vi "Magnet next action.vi"(4 "Overall status in":T2) -> (0 "Overall status Out":T2, 1 "Command out":T1=enum."Set field")   [LabVIEW 2024, in "Magnet module.lvlib"]
doc: "Evaluates next state machine action at the end of regular check.\nIf field is not at desired value, but reached the closest target it sets new target with new ramp."
uses:
  Magnet module.lvlib
  ctl/Overall status.ctl
  ctl/SetField data.ctl
  ctl/Magnet mode public.ctl
  ctl/Actual magnet state.ctl
  ctl/Magnet mode.ctl
  ctl/RampingOutput.ctl
  ctl/Magnet Orders.ctl
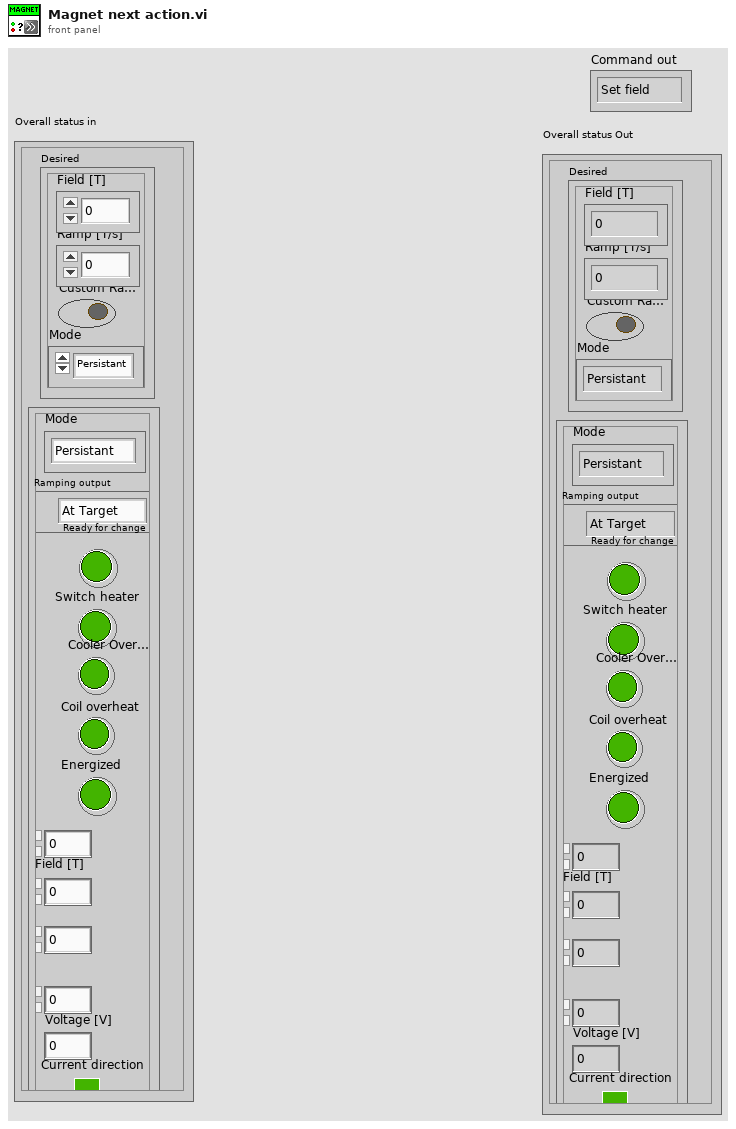
[diagram p1: front panel]
types:
  T1 = typedef "Magnet module.lvlib/Magnet Orders.ctl" = enum16{"Ignore", "Connect", "Update", "Switch mode", "Set field", "Stop ramping", "Equalize output", "Zero output", "Flip polarity", "Blackout", "Set timer", "Eval temperatures", "Disconnect"}
  T2 = typedef "Magnet module.lvlib/Overall status.ctl" = cluster{"Desired":T3, "Actual":T5}
  T3 = typedef "Magnet module.lvlib/SetField data.ctl" = cluster{"Field [T]":dbl, "Ramp [T/s]":dbl, "Custom Ramp?":bool, "Mode":T4}
  T4 = typedef "Magnet module.lvlib/Magnet mode public.ctl" = enum16{"Persistant", "Ramping"}
  T5 = typedef "Magnet module.lvlib/Actual magnet state.ctl" = cluster{"Mode":T6, "Ramping output":T7, "Ready for change":bool, "Switch heater":bool, "Cooler Overheat":bool, "Coil overheat":bool, "Energized":bool, "Output [T]":dbl, "Field [T]":dbl, "Ramp[T/s]":dbl, "Switch\ntemperature [K]":dbl, "Voltage [V]":dbl, "Current direction":bool}
  T6 = typedef "Magnet module.lvlib/Magnet mode.ctl" = enum16{"Persistant", "Switching", "Ramping", "Quenched"}
  T7 = typedef "Magnet module.lvlib/RampingOutput.ctl" = enum16{"At Target", "Go up", "Go down"}
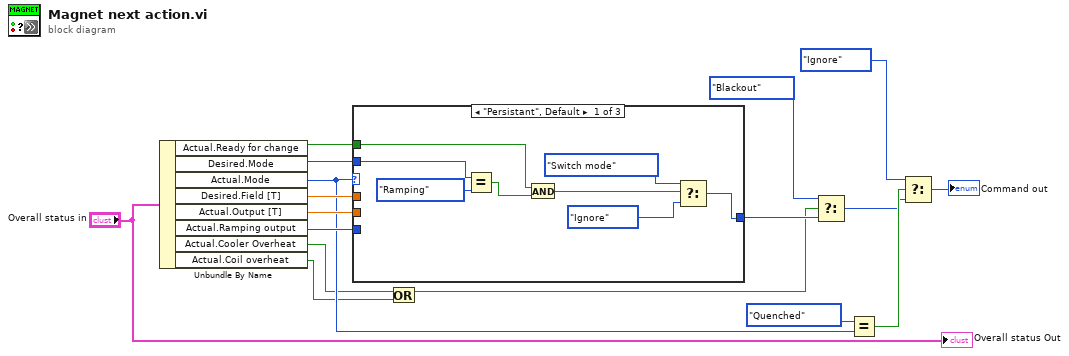
[diagram p0: block diagram]
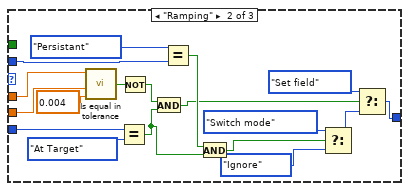
[diagram p2: hidden frame]
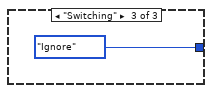
[diagram p3: hidden frame]
diagram:
  n1 = Unbundle By Name("Overall status in") -> ("Actual.Ready for change"=w1:bool, "Desired.Mode"=w4:T4, "Actual.Mode"=w13:T6, "Desired.Field [T]"=w16:dbl, "Actual.Output [T]"=w17:dbl, "Actual.Ramping output"=w15:T7, "Actual.Cooler Overheat"=w7:bool, "Actual.Coil overheat"=w2:bool)
  n2 = case shown="\"Persistant\", Default" w13 {
    tunnel: w17 -> [_ w39 _]
    tunnel: w16 -> [_ w38 _]
    tunnel: [w23 w43 Magnet_Orders."Ignore" ("Command out")] -> w10
    tunnel: w15 -> [_ w35 _]
    tunnel: w4 -> [w21 w34 _]
    tunnel: w1 -> [w18 _ _]
    frame "Persistant", Default {
      n3 = Equal?(x=w21, y=Magnet_mode_public."Ramping" ("Mode")) -> (x = y?=w19:bool)
      n4 = And(x=w18, y=w19) -> (x .and. y?=w22:bool)
      n5 = Select(t=Magnet_Orders."Switch mode" ("Command out"), s=w22, f=Magnet_Orders."Ignore" ("Command out")) -> (s? t:f=w23:T1)
    }
    frame "Ramping" {
      n6 = call "Is equal in tolerance.vi"("Absolut tolerance"=0.004, "Reference value"=w39, "Input value"=w38) -> ("Is in range"=w41:bool)  [unwired: 1 in]
      n7 = Equal?(x=w35, y=RampingOutput."At Target" ("x")) -> (x = y?=w26:bool)
      n8 = Not(x=w41) -> (.not. x?=w40:bool)
      n9 = And(x=w40, y=w26) -> (x .and. y?=w31:bool)
      n10 = Equal?(x=Magnet_mode_public."Persistant" ("Mode"), y=w34) -> (x = y?=w32:bool)
      n11 = And(x=w32, y=w26) -> (x .and. y?=w28:bool)
      n12 = Select(t=Magnet_Orders."Switch mode", s=w28, f=Magnet_Orders."Ignore" ("Command out")) -> (s? t:f=w29:T1)
      n13 = Select(t=Magnet_Orders."Set field" ("Command out"), s=w31, f=w29) -> (s? t:f=w43:T1)
    }
    frame "Switching" {
    }
  }
  n14 = Or(x=w7, y=w2) -> (x .or. y?=w3:bool)
  n15 = Select(t=Magnet_Orders."Blackout", s=w3, f=w10) -> (s? t:f=w5:T1)
  n16 = Equal?(x=Magnet_mode."Quenched", y=w13) -> (x = y?=w11:bool)
  n17 = Select(t=Magnet_Orders."Ignore" ("f"), s=w11, f=w5) -> (s? t:f=→"Command out":T1)
  "Overall status Out" <- "Overall status in"
